vi "GaGe_Timeout.vi"(10 "TimeOut (s)":sgl, 11 "GaGe Handle":T1) -> (2 "String":string, 3 "GaGe Handle Out":T1)   [LabVIEW 2022 SP3]
uses:
  <vilib>/Platform/TimedLoop/XDataNode/XDataNode.xnode
  <vilib>/Platform/TimedLoop/XDataNode/nitl_modes.ctl
  <vilib>/Platform/TimedLoop/XDataNode/XDNodeRunTimeDep.lvlib
  <vilib>/Platform/TimedLoop/XDataNode/wakeup.ctl
  <vilib>/Platform/TimedLoop/XDataNode/timing_clust.ctl
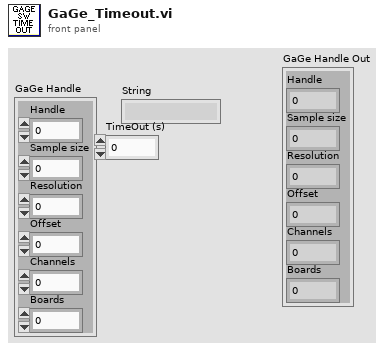
[diagram p1: front panel]
types:
  T1 = cluster{"Handle":u32, "Sample size":u32, "Resolution":i32, "Offset":i32, "Channels":u32, "Boards":u32}
  T2 = typedef "XDNodeRunTimeDep.lvlib/timing_clust.ctl" = cluster{"Expected End [f-1]":u64, "Actual End [f-1]":u64, "Finished Late? [f-1]":bool, "Expected End [i-1]":u64, "Actual End [i-1]":u64, "Finished Late? [i-1]":bool, "Expected Start [i]":u64, "Actual Start [i]":u64, "Expected Start [f]":u64, "Actual Start [f]":u64, "Source Name":string, "Structure Name":string, "Period":i64, "Deadline":i64, "Offset":i64, "Start":i64, "Priority":i32, "Timeout":i32, "Mode":T3, "Wakeup Reason":T4, "Error":errorcluster, "Source Type":string, "Secondary Source Type":string, "Global End Time":u64, "Global Start Time":u64, "Frame Duration":u64, "Iteration Duration":u64, "Assigned CPU":i32, "I/O Scan Engine Mode":u32}
  T3 = typedef "XDNodeRunTimeDep.lvlib/nitl_modes.ctl" = enum32{"No Change", "Process missed periods, maintain original phase", "Discard missed periods, maintain original phase", "Process missed periods, ignore original phase", "Discard missed periods, ignore original phase"}
  T4 = typedef "XDNodeRunTimeDep.lvlib/wakeup.ctl" = enum32{"Normal", "Aborted", "Asynchronous wakeup", "Timing source error", "Timed loop error", "Timeout"}
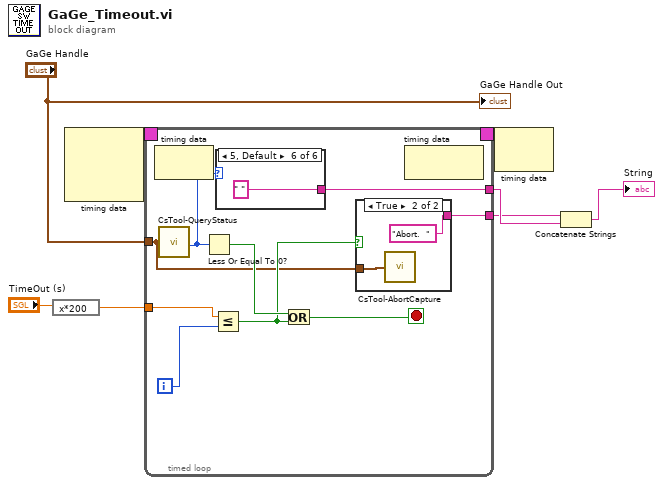
[diagram p0: block diagram]
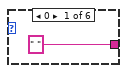
[diagram p3: hidden frame]
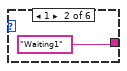
[diagram p4: hidden frame]
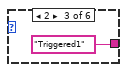
[diagram p5: hidden frame]
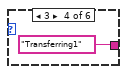
[diagram p6: hidden frame]
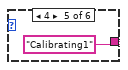
[diagram p7: hidden frame]
diagram:
  n1 = expression code="x*200"("TimeOut (s)") -> (w4:sgl)
  n2 = node-c288() -> (w6:T2)  [unwired: 3 in]
  n3 = timed-loop {
    tunnel: "GaGe Handle" -> [w10]
    tunnel: [w16] -> w3
    timing: w6 -> [_]
    timing-out: [_] -> w5
    tunnel: w4 -> [w13]
    tunnel: [w9] -> w2
    i -> [w14]
    stop <- w12 stop-if-true
    n4 = node-c288() -> ()  [unwired: 1 in, 1 out]
    n5 = call <userlib>:"CsTool-QueryStatus.vi"("Handle Cluster"=w10) -> ("Status"=w17:i32)
    n6 = Less Or Equal To 0?(x=w17) -> (x <= 0?=w15:bool)
    n7 = Less Or Equal?(x=w13, y=w14) -> (x <= y?=w11:bool)
    n8 = case shown="5, Default" w17 {
      tunnel: [" " "Waiting1" "Triggered1" "Transferring1" "Calibrating1" " "] -> w16
      frame 0 {
      }
      frame 1 {
      }
      frame 2 {
      }
      frame 3 {
      }
      frame 4 {
      }
      frame 5, Default {
      }
    }
    n9 = Or(x=w15, y=w11) -> (x .or. y?=w12:bool)
    n10 = case shown="True" w11 {
      tunnel: w10 -> [_ w19]
      tunnel: [_ "Abort.  "] -> w9
      frame False {
      }
      frame True {
        n11 = call <userlib>:"CsTool-AbortCapture.vi"("Handle Cluster"=w19) -> ()  [unwired: 1 out]
      }
    }
    n12 = node-c288() -> ()  [unwired: 1 in, 1 out]
  }
  n13 = node-c288(w5) -> ()  [unwired: 1 out]
  n14 = Concatenate Strings(w2, w3) -> (→"String":string)
  "GaGe Handle Out" <- "GaGe Handle"
